vi "To Tree.vi"(8 "error in (no error)":errorcluster, 10 "Tree Refnum":refnum<vi>, 11 "JSON Datatype in":refnum<class "JSON Datatype.lvclass">=refnum) -> (0 "error out":errorcluster, 3 "JSON Datatype out":refnum<class "JSON Datatype.lvclass">)   [LabVIEW 2017, in "NISE JSON.lvlib" / "JSON Datatype.lvclass"]
uses:
  JSON Datatype.lvclass
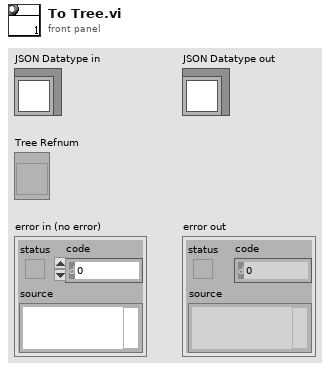
[diagram p1: front panel]
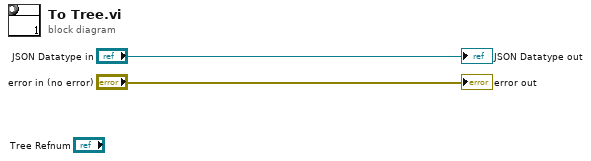
[diagram p0: block diagram]
diagram:
  "error out" <- "error in (no error)"
  "JSON Datatype out" <- "JSON Datatype in"
